vi "ArrowAngleWorking.vi"(7 "error in":errorcluster) -> (20 "Caliper Results (Caliper 1)":sgl[][](array[numeric]) format="%.2f", 27 "error out":errorcluster)   [LabVIEW 2017]
uses:
  <vilib>/vision/NI_Vision_Development_Module.lvlib
panel:
  out "Image Out":T1(plugin-control)
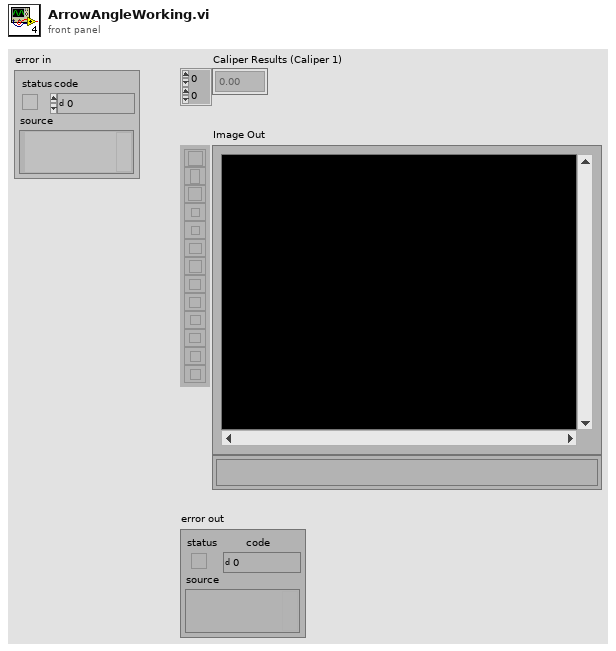
[diagram p1: front panel]
types:
  T1 = typedef "IMAQ Image.ctl" = refnum<image>
  T2 = cluster{"Feature":u32, "Points IDs":cluster{"GUID":string, "Index":i32}[]}[]
  T3 = cluster{"Sigma":sgl, "HThresh":sgl, "LThres":sgl, "WindowSize":i32}
  T4 = cluster{"Number of Matches Requested":i32, "Minimum Match Score":sgl, "Angle Ranges":cluster{"Start Angle":sgl, "End Angle":sgl}[]}
  T5 = cluster{"Global Rectangle":i32[], "Contours":cluster{"ID":enum32{"External", "Internal"}, "Type":u32, "Coordinates":i32[]}[]}
  T6 = typedef "Image Type" = u32
  T7 = cluster{"Position":cluster{"x":sgl, "y":sgl}, "Angle":sgl, "Scale":sgl, "Score":sgl, "Bounding Box":cluster{"x":sgl, "y":sgl}[]}[]
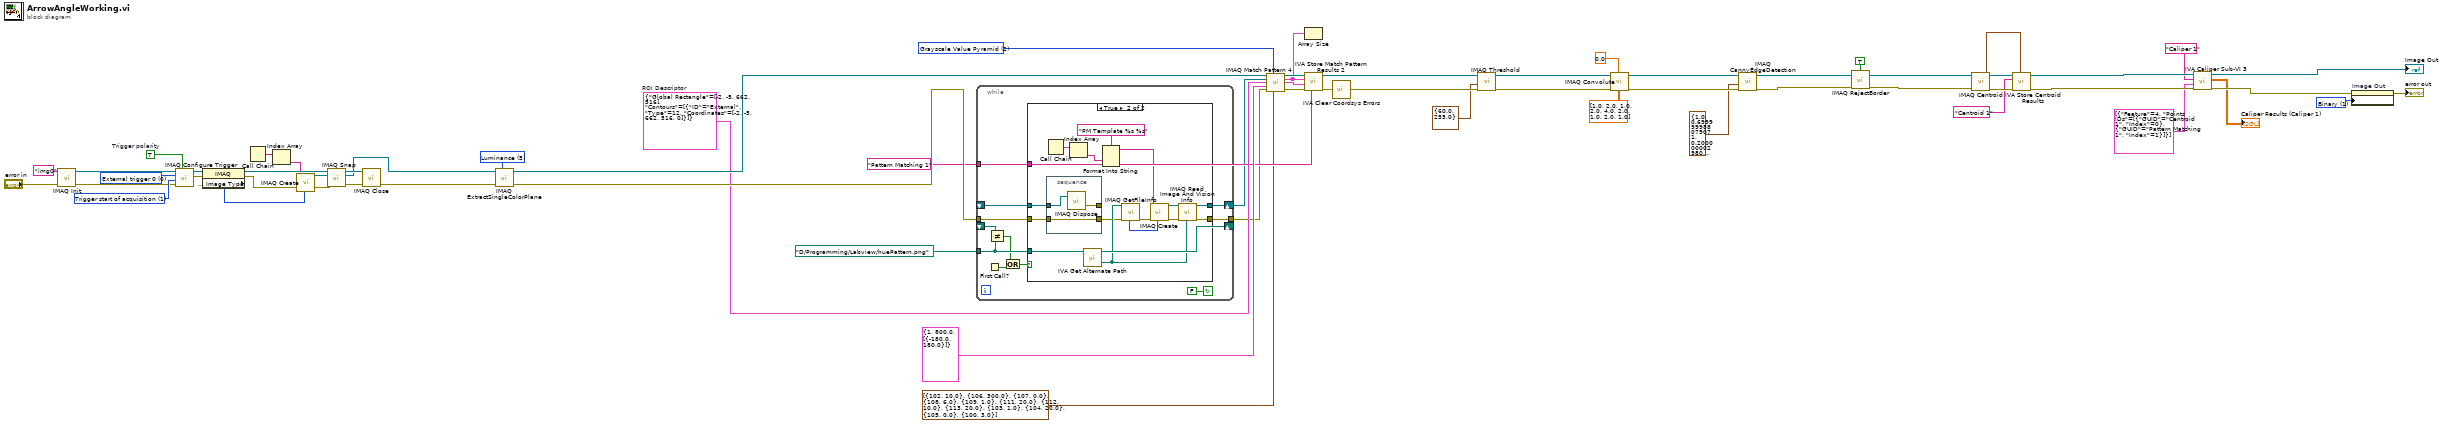
[diagram p0: block diagram]
diagram:
  w1 = u32 1 items=["Grayscale", "Binary", "Gradient", "Rainbow", "Temperature", "User Defined", "Binary 16 Bit", "Gradient 16 Bit", "Rainbow 16 Bit", "Temperature 16 Bit", "User Defined 16 Bit"] ("Palette Type")
  w37 = 2 items=["All", "Low Discrepancy Sampling", "Grayscale Value Pyramid", "Gradients Pyramid"] ("Algorithm")
  w34 = "Pattern Matching 1" ("Step Name")
  w36 = T5 {"Global Rectangle"=[-2, -5, 662, 516], "Contours"=[{"ID"=enum."External", "Type"=12, "Coordinates"=[-2, -5, 662, 516, 0]}]}  # ROI Descriptor
  w44 = 5 items=["Red", "Green", "Blue", "Hue", "Saturation", "Luminance", "Value", "Intensity"] ("Color Plane")
  w56 = u32 1 items=["Disabled", "Trigger start of acquisition", "Trigger start of each buffer list", "Trigger each buffer", "Trigger each line (linescan)"] ("Trigger action")
  w57 = u32 0 items=["External trigger 0", "External trigger 1", "External trigger 2", "External trigger 3", "RTSI line 0", "RTSI line 1", "RTSI line 2", "RTSI line 3", "RTSI line 4", "RTSI line 5", "RTSI line 6"] ("Trigger line")
  w58 = TRUE  # Trigger polarity
  n1 = call <vilib>:"IMAQ Init.vi"("error in (no error)"="error in", "Interface Name"="img0") -> ("error out"=w55:errorcluster, "IMAQ Session Out"=w59:refnum<k11>)  [unwired: 8 out]
  n2 = call <vilib>:"IMAQ Configure Trigger.vi"("Trigger polarity"=w58, "error in (no error)"=w55, "Trigger action"=w56, "Trigger line"=w57, "IMAQ Session In"=w59) -> ("error out"=w53:errorcluster, "IMAQ Session Out"=w54:refnum<k11>)  [unwired: 2 in, 3 out]
  n3 = property class="IMAQ"(reference=w54, error in=w53) -> (reference out=w52:refnum<k11>, error out=w51:errorcluster, "Image Parameters : Image Type"=w50:u32)
  n4 = Call Chain() -> (call chain=w46:string[])
  n5 = Index Array(array=w46) -> (element=w45:string)  [unwired: 1 in]
  n6 = call "IMAQ Create"("Image Name"=w45, "Image Type"=w50, "error in (no error)"=w51) -> ("New Image"=w49:T1, "error out"=w48:errorcluster)  [unwired: 1 in, 1 out]
  n7 = call <vilib>:"IMAQ Snap.vi"("error in (no error)"=w48, "Image In"=w49, "IMAQ Session In"=w52) -> ("error out"=w61:errorcluster, "Image Out"=w43:T1, "IMAQ Session Out"=w62:refnum<k11>)  [unwired: 6 out]
  n8 = call <vilib>:"IMAQ Close.vi"("error in (no error)"=w61, "IMAQ Session In"=w62) -> ("error out"=w60:errorcluster)  [unwired: 9 out]
  n9 = call "IMAQ ExtractSingleColorPlane"("Color Plane"=w44, "error in (no error)"=w60, "Image Src"=w43) -> ("error out"=w42:errorcluster, "Image Dst Out"=w40:T1)  [unwired: 1 in, 6 out]
  n10 = while {
    shift-right: [w74] -> w31
    shift-left: _ -> [w73]
    tunnel: [w71] -> w30
    tunnel: w42 -> [w70]
    tunnel: path "D:/Programming/Labview/huePattern.png" ("Template File Path") -> [w67]
    tunnel: w34 -> [w69]
    shift-right: [w67] -> _
    shift-left: _ -> [w68]
    stop <- FALSE continue-if-true
    n11 = First Call?() -> (First Call?: T/F=w66:bool)
    n12 = Not Equal?(x=w68, y=w67) -> (x != y?=w65:bool)
    n13 = Or(x=w65, y=w66) -> (x .or. y?=w64:bool)
    n14 = case shown="True" w64 {
      tunnel: [w76 w90] -> w74
      tunnel: w73 -> [w76 w82]
      tunnel: [w75 w87] -> w71
      tunnel: w70 -> [w75 w81]
      tunnel: w67 -> [_ w83]
      tunnel: w69 -> [_ w84]
      frame False {
      }
      frame True {
        n15 = stacked-sequence {
          tunnel: w82 -> [w95]
          tunnel: w81 -> [w94]
          tunnel: [w94] -> w77
          tunnel: [w93] -> _
          frame #0 {
            n16 = call "IMAQ Dispose"("Image"=w95) -> ("error out"=w93:errorcluster)  [unwired: 2 in, 3 out]
          }
        }
        n17 = Call Chain() -> (call chain=w86:string[])
        n18 = Index Array(array=w86) -> (element=w85:string)  [unwired: 1 in]
        n19 = call <vilib>:"IVA Get Alternate Path.vi"("Path In"=w83) -> ("Path Out"=w79:path)  [unwired: 10 out]
        n20 = Format Into String(format string="PM Template %s %s" ("Image Name"), w85, w84) -> (resulting string=w92:string)  [unwired: 2 in, 1 out]
        n21 = call "IMAQ GetFileInfo"("error in (no error)"=w77, "File Path"=w79) -> ("error out"=w78:errorcluster, "Image Type"=w80:T6)  [unwired: 3 in, 5 out]
        n22 = call "IMAQ Create"("Image Name"=w92, "Image Type"=w80, "error in (no error)"=w78) -> ("New Image"=w89:T1, "error out"=w88:errorcluster)  [unwired: 1 in, 1 out]
        n23 = call "IMAQ Read Image And Vision Info"("File Path"=w79, "error in (no error)"=w88, "Image"=w89) -> ("error out"=w87:errorcluster, "Image Out"=w90:T1)  [unwired: 1 in, 6 out]
      }
    }
  }
  n24 = call "IMAQ Match Pattern 4"("Image"=w40, "Algorithm"=w37, "Template Image"=w31, "ROI Descriptor"=w36, "Parameters"=T4 {"Number of Matches Requested"=1, "Minimum Match Score"=800.0, "Angle Ranges"=[{"Start Angle"=-180.0, "End Angle"=180.0}]}, "error in (no error)"=w30, "Advanced Options"=cluster{"Item":u16, "Value":dbl}[] [{"Item"=102, "Value"=10.0}, {"Item"=106, "Value"=300.0}, {"Item"=107, "Value"=0.0}, {"Item"=108, "Value"=6.0}, {"Item"=109, "Value"=1.0}, {"Item"=111, "Value"=20.0}, {"Item"=112, "Value"=10.0}, {"Item"=113, "Value"=20.0}, {"Item"=103, "Value"=1.0}, {"Item"=104, "Value"=20.0}, {"Item"=105, "Value"=0.0}, {"Item"=100, "Value"=3.0}]) -> ("Image (duplicate)"=w38:T1, "Matches (pixel)"=w33:T7, "Matches (real-world)"=w32:T7, "error out"=w39:errorcluster)  [unwired: 4 in, 1 out]
  n25 = Array Size(array=w33) -> ()  [unwired: 1 out]
  n26 = call <vilib>:"IVA Store Match Pattern Results 2.vi"("Step Name"=w34, "error in (no error)"=w39, "Matches (real-world)"=w32, "Matches (pixel)"=w33, "Image in"=w38) -> ("error out"=w29:errorcluster, "Image dup"=w25:T1)  [unwired: 1 in, 4 out]
  n27 = call <vilib>:"IVA Clear Coordsys Errors.vi"("error in (no error)"=w29) -> ("error out"=w28:errorcluster)  [unwired: 10 in]
  n28 = call "IMAQ Threshold"("error in (no error)"=w28, "Range"=cluster{"Lower value":sgl, "Upper value":sgl} {"Lower value"=60.0, "Upper value"=255.0}, "Image Src"=w25) -> ("error out"=w24:errorcluster, "Image Dst Out"=w22:T1)  [unwired: 3 in, 4 out]
  n29 = call "IMAQ Convolute"("Kernel"=sgl[][] [[1.0, 2.0, 1.0], [2.0, 4.0, 2.0], [1.0, 2.0, 1.0]], "Divider (kernel sum)"=sgl 0.0 ("Divider"), "error in (no error)"=w24, "Image Src"=w22) -> ("error out"=w21:errorcluster, "Image Dst Out"=w19:T1)  [unwired: 3 in, 3 out]
  n30 = call "IMAQ CannyEdgeDetection"("Image Src"=w19, "Filter Parameters"=T3 {"Sigma"=1.0, "HThresh"=0.7, "LThres"=0.2, "WindowSize"=9}, "error in (no error)"=w21) -> ("Image Dst Out"=w15:T1, "error out"=w18:errorcluster)  [unwired: 1 in, 4 out]
  n31 = call "IMAQ RejectBorder"("error in (no error)"=w18, "Image Src"=w15, "Connectivity 4/8 (8)"=TRUE) -> ("error out"=w14:errorcluster, "Image Dst Out"=w11:T1)  [unwired: 1 in, 2 out]
  n32 = call "IMAQ Centroid"("error in (no error)"=w14, "Image"=w11) -> ("error out"=w13:errorcluster, "Centroid"=w9:cluster{"X Centroid":sgl, "Y Centroid":sgl})  [unwired: 1 in, 1 out]
  n33 = call <vilib>:"IVA Store Centroid Results.vi"("Centroid in"=w9, "error in (no error)"=w13, "Step Name"="Centroid 1", "Image in"=w11) -> ("error out"=w12:errorcluster, "Image dup"=w8:T1)  [unwired: 6 out]
  n34 = call <vilib>:"IVA Caliper Sub-VI 3.vi"("error in"=w12, "Parameters"=T2 [{"Feature"=4, "Points IDs"=[{"GUID"="Centroid 1", "Index"=0}, {"GUID"="Pattern Matching 1", "Index"=1}]}], "Step Name"="Caliper 1", "Image In"=w8) -> ("error out"=w7:errorcluster, "Results (Pixels)"=→"Caliper Results (Caliper 1)":sgl[][], "Image Out"=→"Image Out":T1)  [unwired: 1 in, 4 out]
  n35 = property on="Image Out" class="ImageControl"(error in=w7, "Palette:Palette Type"=w1) -> (error out=→"error out":errorcluster)  [unwired: 1 in, 1 out]
